vi "Reentrant FGV Test.vi"() -> ()   [LabVIEW 2014]
uses:
  Controls/Drone Information.ctl
  Controls/Base Mode.ctl
  Controls/Aircraft Mode.ctl
  Telemetry/Controls/Telemetry Connection Type.ctl
  Set Aircraft Information.vi
  Get Aircraft Information.vi
panel:
  out "Aircraft Information Out":T1={"Heart Beat"=FALSE, "Aircraft ID"=0, "Downlink Port"="", "Tag ID"="", "System Status"="", "Base Mode"={"Custom Mode"=FALSE, "Test Enabled"=FALSE, "Autonomous Mode"=FALSE, "Guided Mode"=FALSE, "Stabilization Enabled"=FALSE, "HIL Enabled"=FALSE, "Manual Mode"=FALSE, "Arm"=FALSE}, "Armed/Disarmed"=FALSE, "Battery Voltage"=0.0, "Control Mode"=enum."Stabalise", "Initialisation"=0, "Heart Beat Status"=FALSE, "Uplink Port"="", "UDP connection ID"=refnum, "Connection Type"=enum."Serial", "Mode"="", "UDP IP Address"="", "Mission Uploaded"=FALSE} {"Initialisation" scale=0.0..100.0}
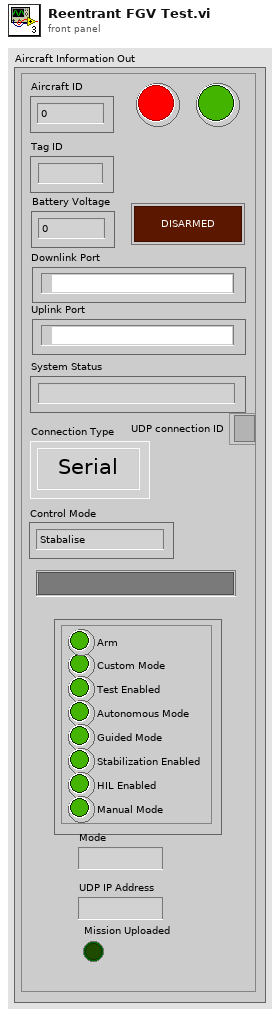
[diagram p1: front panel]
types:
  T1 = typedef "Drone Information.ctl" = cluster{"Heart Beat":bool, "Aircraft ID":u8, "Downlink Port":refnum<visa-resource-name>, "Tag ID":string, "System Status":string, "Base Mode":T2, "Armed/Disarmed":bool, "Battery Voltage":dbl, "Control Mode":T3, "Initialisation":u8, "Heart Beat Status":bool, "Uplink Port":refnum<visa-resource-name>, "UDP connection ID":refnum<k16>, "Connection Type":T4, "Mode":string, "UDP IP Address":string, "Mission Uploaded":bool}
  T2 = typedef "Base Mode.ctl" = cluster{"Custom Mode":bool, "Test Enabled":bool, "Autonomous Mode":bool, "Guided Mode":bool, "Stabilization Enabled":bool, "HIL Enabled":bool, "Manual Mode":bool, "Arm":bool}
  T3 = typedef "Aircraft Mode.ctl" = enum16{"Loiter", "Stabalise", "Failsafe", "Emergency Stop"}
  T4 = typedef "Telemetry Connection Type.ctl" = enum16{"Serial", "UDP", "TCP"}
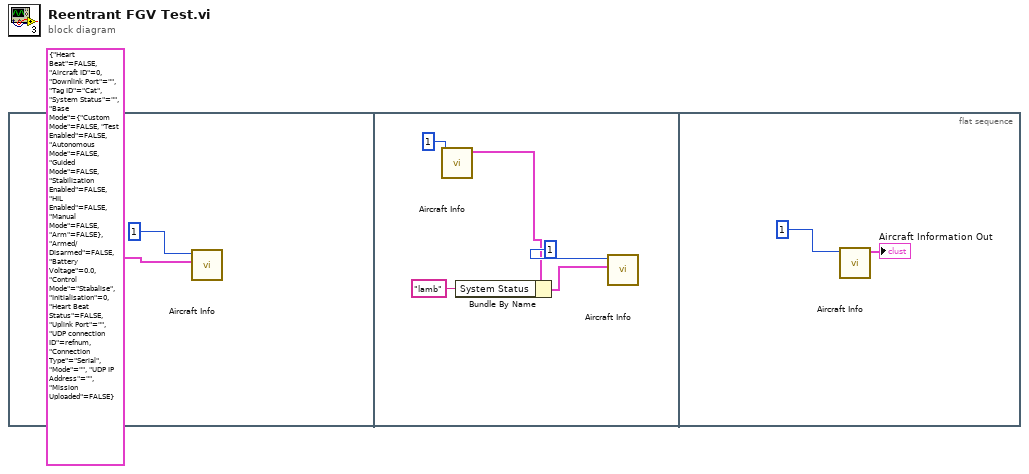
[diagram p0: block diagram]
diagram:
  n1 = flat-sequence {
    frame #0 {
      n2 = call-poly "Aircraft Info.vi"("Aircraft Information In"=T1 {"Heart Beat"=FALSE, "Aircraft ID"=0, "Downlink Port"="", "Tag ID"="Cat", "System Status"="", "Base Mode"={"Custom Mode"=FALSE, "Test Enabled"=FALSE, "Autonomous Mode"=FALSE, "Guided Mode"=FALSE, "Stabilization Enabled"=FALSE, "HIL Enabled"=FALSE, "Manual Mode"=FALSE, "Arm"=FALSE}, "Armed/Disarmed"=FALSE, "Battery Voltage"=0.0, "Control Mode"=enum."Stabalise", "Initialisation"=0, "Heart Beat Status"=FALSE, "Uplink Port"="", "UDP connection ID"=refnum, "Connection Type"=enum."Serial", "Mode"="", "UDP IP Address"="", "Mission Uploaded"=FALSE}, "Aircraft ID"=u8 1) -> ()  [unwired: 9 in, 1 out]
    }
    frame #1 {
      n3 = call-poly "Aircraft Info.vi"("Aircraft ID"=u8 1) -> ("Aircraft Information Out"=w5:T1)  [unwired: 9 in, 1 out]
      n4 = Bundle By Name(cluster=w5, "System Status"="lamb") -> (w3:T1)
      n5 = call-poly "Aircraft Info.vi"("Aircraft Information In"=w3, "Aircraft ID"=u8 1) -> ()  [unwired: 9 in, 1 out]
    }
    frame #2 {
      n6 = call-poly "Aircraft Info.vi"("Aircraft ID"=u8 1) -> ("Aircraft Information Out"=→"Aircraft Information Out":T1)  [unwired: 9 in, 1 out]
    }
  }
